vi "imaq save GEECS.vi"(7 "Status":T2, 8 "error in (no error)":errorcluster, 9 "file already written":bool, 10 "Refnum in":T1, 11 "FakeCamera in":refnum<class "Point Grey Camera.lvclass">) -> (0 "error out":errorcluster, 3 "FakeCamera out":refnum<class "Point Grey Camera.lvclass">)   [LabVIEW 2020, in "Point Grey Camera.lvclass"]
uses:
  Point Grey Camera.lvclass
  Image save type.ctl
  1st or last shot of scan.ctl
  IMAQ Image.ctl
  Point Grey Camera.lvclass/Point Grey Camera.ctl
panel:
  out "Save type":T3
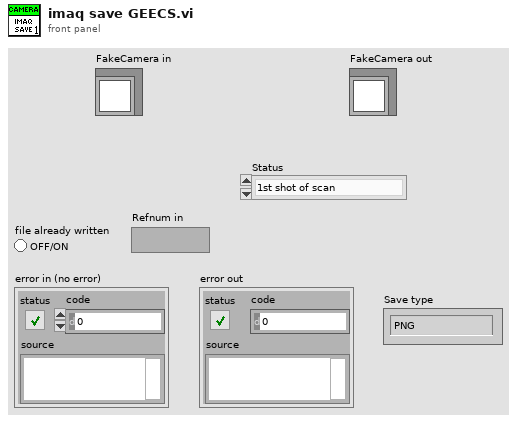
[diagram p1: front panel]
types:
  T1 = typedef "IMAQ Image.ctl" = refnum<image>
  T2 = typedef "1st or last shot of scan.ctl" = enum16{"1st shot of scan", "1st shot after scan end", "other"}
  T3 = typedef "Image save type.ctl" = enum16{"PNG", "BMP", "JPEG", "TDMS", "hdf5"}
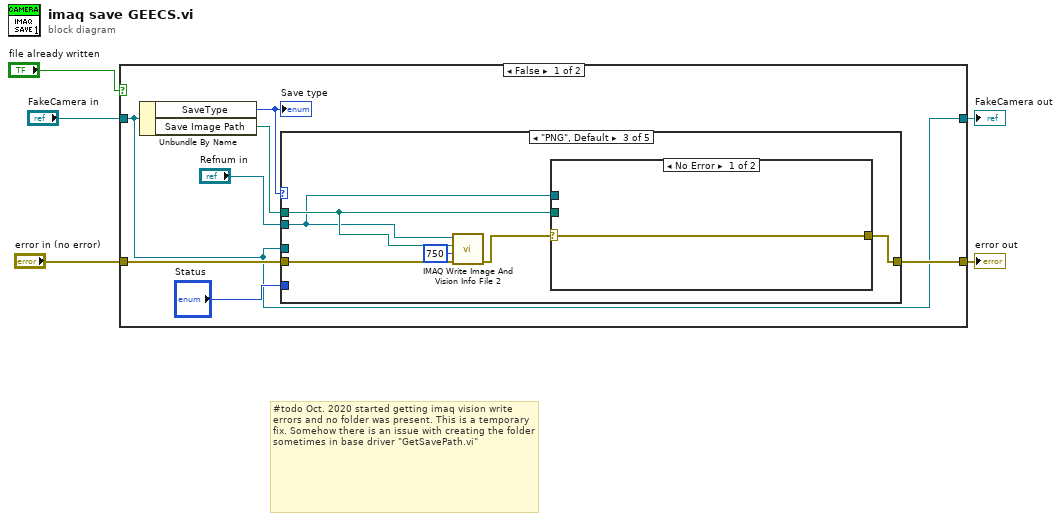
[diagram p0: block diagram]
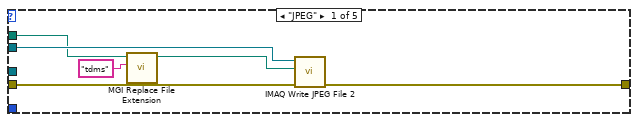
[diagram p2: hidden frame]
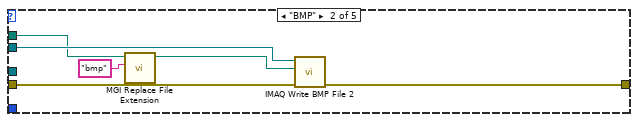
[diagram p3: hidden frame]
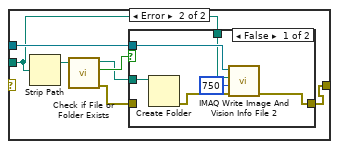
[diagram p4: hidden frame]
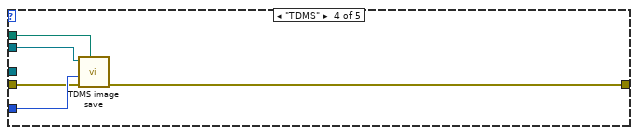
[diagram p6: hidden frame]
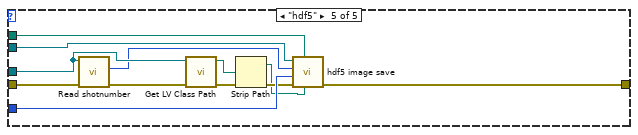
[diagram p7: hidden frame]
diagram:
  # "#todo Oct. 2020 started getting imaq vision write errors and no folder was present. This is a temporary fix. Somehow there is an issue with creating the folder sometimes in base driver \"GetSavePath.vi\""
  n1 = case shown="False" "file already written" {
    tunnel: [w12 w63] -> w5
    tunnel: "error in (no error)" -> [w7 w63]
    tunnel: [w6 w62] -> w2
    tunnel: "FakeCamera in" -> [w6 w62]
    frame False {
      n2 = Unbundle By Name(w6) -> ("SaveType"=w9:T3, "Save Image Path"=w11:path)
      "Save type" <- w9
      n3 = case shown="\"PNG\", Default" w9 {
        tunnel: w7 -> [w18 w24 w30 w47 w55]
        tunnel: "Refnum in" -> [w16 w22 w25 w46 w58]
        tunnel: w11 -> [w13 w20 w26 w50 w61]
        tunnel: [w15 w19 w27 w49 w60] -> w12
        tunnel: "Status" -> [_ _ _ w48 w59]
        tunnel: w6 -> [_ _ _ _ w56]
        frame "JPEG" {
          n4 = call "MGI Replace File Extension.vi"("New Extension (txt)"="tdms", "Path In"=w13) -> ("Path Out"=w17:path)  [unwired: 8 in, 1 out]
          n5 = call "IMAQ Write JPEG File 2"("error in (no error)"=w18, "File Path"=w17, "Image"=w16) -> ("error out"=w15:errorcluster)  [unwired: 7 in, 1 out]
        }
        frame "BMP" {
          n6 = call "MGI Replace File Extension.vi"("New Extension (txt)"="bmp", "Path In"=w20) -> ("Path Out"=w23:path)  [unwired: 8 in, 1 out]
          n7 = call "IMAQ Write BMP File 2"("error in (no error)"=w24, "File Path"=w23, "Image"=w22) -> ("error out"=w19:errorcluster)  [unwired: 7 in, 1 out]
        }
        frame "PNG", Default {
          n8 = call "IMAQ Write Image And Vision Info File 2"("error in (no error)"=w30, "Image Quality"=u32 750, "File Path"=w26, "Image"=w25) -> ("error out"=w28:errorcluster)  [unwired: 6 in, 1 out]
          n9 = case shown="No Error" w28 {
            selector: w28 -> [w31 _]
            tunnel: [w31 w33] -> w27
            tunnel: w26 -> [_ w32]
            tunnel: w25 -> [_ w34]
            frame No Error {
            }
            frame Error {
              n10 = Strip Path(path=w32) -> (stripped path=w38:path)  [unwired: 1 out]
              n11 = call "Check if File or Folder Exists.vi"("path"=w38) -> ("error out"=w35:errorcluster, "file or folder exists?"=w37:bool, "dup path"=w36:path)  [unwired: 1 in, 7 out]
              n12 = case shown="False" w37 {
                tunnel: w36 -> [w44 _]
                tunnel: [w40 w45] -> w33
                tunnel: w35 -> [_ w45]
                tunnel: w34 -> [w42 _]
                tunnel: w32 -> [w39 _]
                frame False {
                  n13 = Create Folder(path (use dialog)=w44) -> (error out=w41:errorcluster)  [unwired: 1 in, 3 out]
                  n14 = call "IMAQ Write Image And Vision Info File 2"("error in (no error)"=w41, "Image Quality"=u32 750, "File Path"=w39, "Image"=w42) -> ("error out"=w40:errorcluster)  [unwired: 6 in, 1 out]
                }
                frame True {
                }
              }
            }
          }
        }
        frame "TDMS" {
          n15 = call "TDMS image save.vi"("Save Image Path"=w50, "error in (no error)"=w47, "Status"=w48, "Refnum in"=w46) -> ("error out"=w49:errorcluster)  [unwired: 7 in]
        }
        frame "hdf5" {
          n16 = call-dynamic "Read shotnumber.vi"("error in (no error)"=w55, "BaseDriver in"=w56) -> ("error out"=w53:errorcluster, "shotnumber"=w54:i32)  [unwired: 6 in, 2 out]
          n17 = call "Get LV Class Path.vi"("error in (no error)"=w53, "object"=w56) -> ("error out"=w57:errorcluster, "class path"=w52:path)  [unwired: 8 in]
          n18 = Strip Path(path=w52) -> (stripped path=w51:path)  [unwired: 1 out]
          n19 = call "hdf5 image save.vi"("class path"=w51, "Save Image Path"=w61, "error in (no error)"=w57, "Status"=w59, "image #"=w54, "Refnum in"=w58) -> ("error out"=w60:errorcluster)  [unwired: 5 in]
        }
      }
    }
    frame True {
    }
  }
  "error out" <- w5
  "FakeCamera out" <- w2
